vi "Algae Immediate.vi"(0 "Operation":T2, 1 "Algae State":T1=enum."Intake Algae", 2 "Setpoint":dbl, 3 "Command Info In":T3, 4 "Description":string, 5 "Negate or Confirm?":bool) -> (10 "Command Info Out":T3)   [LabVIEW 2023]
doc: "This template is useful for immediate subsystem actions that do not need deadband filtering\n\nBe sure to right-click and select New from Template and save with a new command name."
uses:
  <vilib>/Rock Robotics/WPI/Framework/Command Status Info.ctl
  <vilib>/Rock Robotics/WPI/Framework/Completion Status.ctl
  <vilib>/Rock Robotics/WPI/Framework/Completion Notifier.ctl
  Implementation/Algae Operations.ctl
  Support Code/Teleop Util/Algae States.ctl
  Implementation/Algae Setpoints.ctl
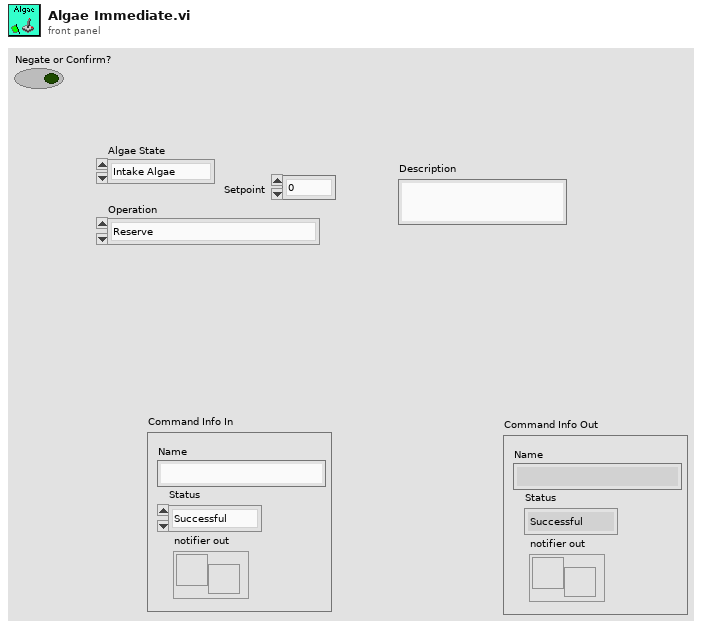
[diagram p1: front panel]
types:
  T1 = typedef "Algae States.ctl" = enum16{"Idle", "Intake Algae", "Outtake Algae", "Stow", "Manual Overrides", "Fling"}
  T2 = typedef "Algae Operations.ctl" = enum16{"Reserve", "Read Current", "Immediate", "Calibrate"}
  T3 = typedef "Command Status Info.ctl" = cluster{"Name":string, "Status":T4, "notifier out":T5}
  T4 = typedef "Completion Status.ctl" = enum16{"Successful", "Aborted", "Incomplete"}
  T5 = typedef "Completion Notifier.ctl" = refnum<notifier>
  T6 = typedef "Algae Setpoints.ctl" = cluster{"Operation":T2, "Setpoint":dbl, "Duration":dbl, "Algae State":T1, "Negate or Confirm?":bool}
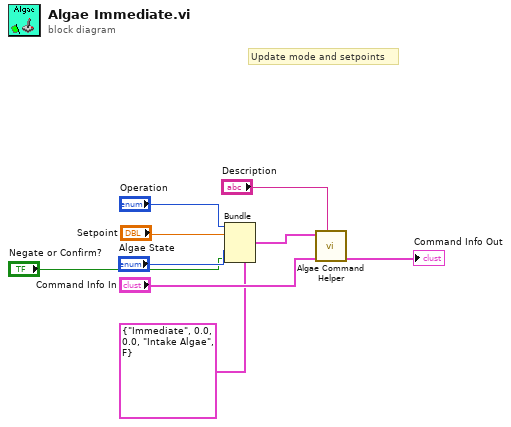
[diagram p0: block diagram]
diagram:
  # "Update mode and setpoints"
  n1 = Bundle(cluster=T6 {"Operation"=enum."Immediate", "Setpoint"=0.0, "Duration"=0.0, "Algae State"=enum."Intake Algae", "Negate or Confirm?"=FALSE} ("SubSystem Data"), "Operation"="Operation", "Setpoint"="Setpoint", "Algae State"="Algae State", "Negate or Confirm?"="Negate or Confirm?") -> (w4:T6)  [unwired: 1 in]
  n2 = call "Algae Command Helper.vi"("Description"="Description", "Command Info In"="Command Info In", "SubSystem Data"=w4) -> ("Command Info Out"=→"Command Info Out":T3)  [unwired: 6 in, 2 out]
